vi "MX100 Example.vi"() -> ()   [LabVIEW 2016]
uses:
  Type Definitions/MX100 Initialization.ctl
  Type Definitions/MX100 Data.ctl
panel:
  out "Loop Count":i32
  in  "stop":bool
  out "MX100 Cluster Out":T1={"Base Time"=0, "Session Number"=0, "Last Data Number"={"High"=-1, "Low"=4294967295}, "Channel List"=[], "FIFO Number (0)"=0, "Channel Number (1)"=1, "Select FIFO or Channel (F:Channel)"=FALSE, "MX100 Data"={"Measurement Values out"=[], "Date/Time"=""}} {"Channel Number (1)" min=1 max=60 step=1; "FIFO Number (0)" min=-1 max=2 step=1}
  in  "Host Address (\"192.168.1.1\")":string="172.16.90.100"
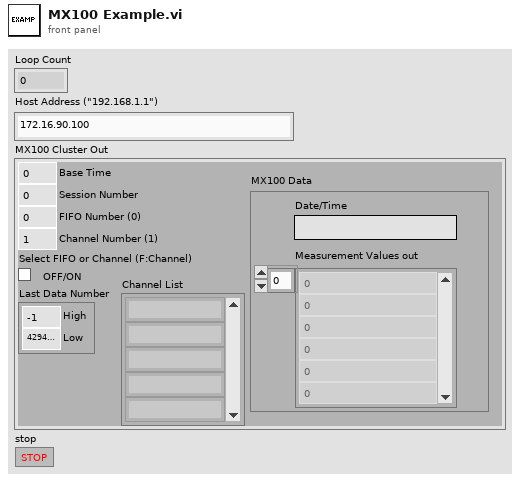
[diagram p1: front panel]
types:
  T1 = typedef "MX100 Initialization.ctl" = cluster{"Base Time":i32, "Session Number":i32, "Last Data Number":cluster{"High":i32, "Low":u32}, "Channel List":string[], "FIFO Number (0)":i32, "Channel Number (1)":i32, "Select FIFO or Channel (F:Channel)":bool, "MX100 Data":T2}
  T2 = typedef "MX100 Data.ctl" = cluster{"Measurement Values out":dbl[], "Date/Time":string}
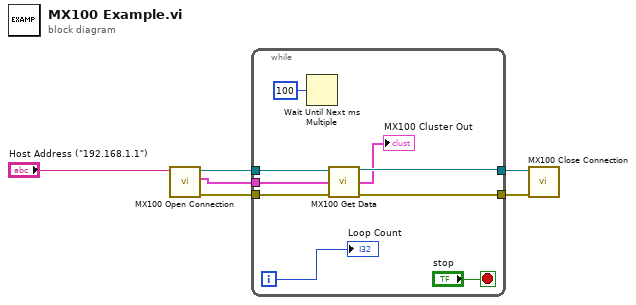
[diagram p0: block diagram]
diagram:
  n1 = call "MX100 Open Connection.vi"("Host Address (\"192.168.1.1\")"="Host Address (\"192.168.1.1\")") -> ("error out"=w2:errorcluster, "MX100 Cluster"=w1:T1, "VISA Refnum out"=w5:refnum<visa-resource-name>)  [unwired: 8 in]
  n2 = while {
    tunnel: w1 -> [w11]
    tunnel: w5 -> [w15]
    tunnel: [w14] -> w4
    tunnel: w2 -> [w12]
    tunnel: [w13] -> w3
    i -> [w7]
    stop <- "stop" stop-if-true
    n3 = Wait Until Next ms Multiple(millisecond multiple=u32 100) -> ()  [unwired: 1 out]
    n4 = call "MX100 Get Data.vi"("VISA Refnum in"=w15, "MX100 Cluster In"=w11, "error in (no error)"=w12) -> ("VISA Refnum out"=w14:refnum<visa-resource-name>, "MX100 Cluster Out"=→"MX100 Cluster Out":T1, "error out"=w13:errorcluster)  [unwired: 10 in]
    "Loop Count" <- w7
  }
  n5 = call "MX100 Close Connection.vi"("error in (no error)"=w3, "VISA Refnum in"=w4) -> ()  [unwired: 9 in, 1 out]
